vi "Build Packet Header.vi"(9 "Length":i32, 10 "TAI Time (ns)":i64, 11 "pcap Parse and Build in":refnum<class "pcap_Parse_Build_CIF.lvclass">) -> (2 "Flattened Data out":u8[](array[numeric])=[0, 0, 0, 0, 0, 0, 0, 0, 1, 2, 3, 4, 5], 3 "pcap Parse and Build out":refnum<class "pcap_Parse_Build_CIF.lvclass">)   [LabVIEW 2021, in "pcap_Parse_Build_CIF.lvclass"]
uses:
  pcap_Parse_Build_CIF.lvclass
  Typedef/Packet Header.ctl
  pcap_Parse_Build_CIF.lvclass/pcap_Parse_Build_CIF.ctl
  <vilib>/CIF Foundation/CIF Utilities/DataTypes/Flatten Unflatten/Flatten U32.vi
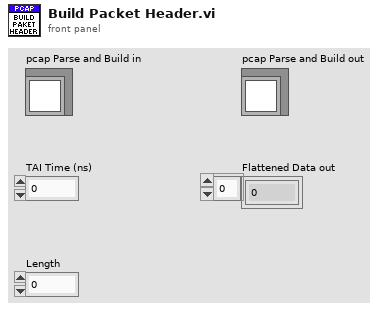
[diagram p1: front panel]
types:
  T1 = typedef "pcap_Parse_Build_CIF.lvclass/Packet Header.ctl" = cluster{"Timestamp (s)":u32, "Timestamp (ns)":u32, "Inc Length":u32, "Orig Length":u32}
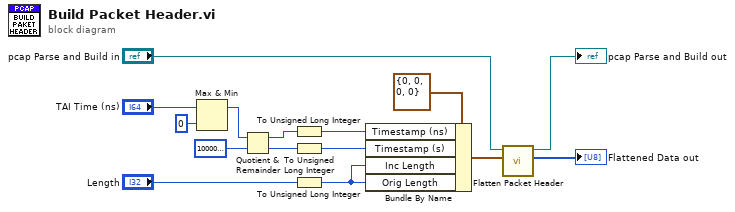
[diagram p0: block diagram]
diagram:
  n1 = Max & Min(x="TAI Time (ns)", y=i64 0) -> (max(x,y)=w9:i64)  [unwired: 1 out]
  n2 = Quotient & Remainder(x=w9, y=i64 1000000000) -> (x-y*floor(x/y)=w13:i64, floor(x/y)=w12:i64)
  n3 = To Unsigned Long Integer(number=w13) -> (unsigned 32bit integer=w8:u32)
  n4 = To Unsigned Long Integer(number=w12) -> (unsigned 32bit integer=w7:u32)
  n5 = To Unsigned Long Integer(number="Length") -> (unsigned 32bit integer=w15:u32)
  n6 = Bundle By Name(cluster=T1 {"Timestamp (s)"=0, "Timestamp (ns)"=0, "Inc Length"=0, "Orig Length"=0} ("Packet Header in"), "Timestamp (ns)"=w8, "Timestamp (s)"=w7, "Inc Length"=w15, "Orig Length"=w15) -> (w4:T1)
  n7 = call "Flatten Packet Header.vi"("Packet Header in"=w4, "pcap Parse and Build in"="pcap Parse and Build in") -> ("Flattened Data out"=→"Flattened Data out":u8[], "pcap Parse and Build out"=→"pcap Parse and Build out":refnum<class "pcap_Parse_Build_CIF.lvclass">)  [unwired: 8 in]
